vi "Set Pending Transfers.vi"(8 "error in":errorcluster, 10 "Pending IResponse":refnum<data-value>, 11 "SDO Manager Worker in":refnum<class "Response Matcher.lvclass">) -> (0 "error out":errorcluster, 3 "SDO Manager Worker out":refnum<class "Response Matcher.lvclass">)   [LabVIEW 2020, in "CANopen.lvlib" / "Response Matcher.lvclass"]
uses:
  Response Matcher.lvclass
  IResponse/IMatch Response.lvclass
  Response Matcher.lvclass/Response Matcher.ctl
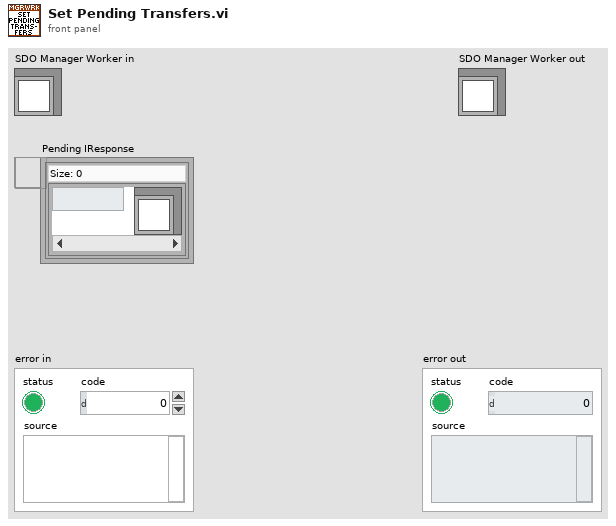
[diagram p1: front panel]
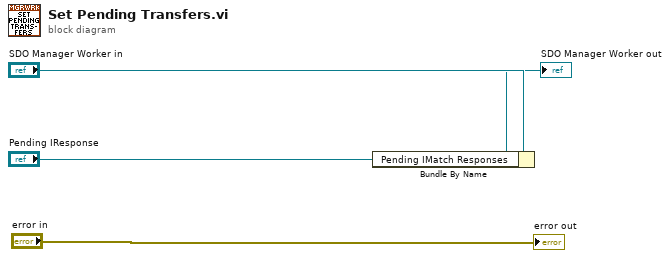
[diagram p0: block diagram]
diagram:
  n1 = Bundle By Name(cluster="SDO Manager Worker in", "Pending IMatch Responses"="Pending IResponse") -> (→"SDO Manager Worker out":refnum<class "Response Matcher.lvclass">)
  "error out" <- "error in"
